vi "Get Position.vi"(8 "error in":errorcluster, 11 "Cell Context in":refnum<class "Cell Context.lvclass">) -> (0 "error out":errorcluster, 2 "Position":cluster{"Row":i32, "Column":i32}, 3 "Cell Context out":refnum<class "Cell Context.lvclass">)   [LabVIEW 2023, in "SourceGrid.lvlib" / "Cell Context.lvclass"]
uses:
  Cell Context.lvclass
  Cell Context.lvclass/Cell Context.ctl
  D:/git/Sourcegrid-LabVIEW/dll/SourceGrid.dll
  dll/SourceGrid.dll
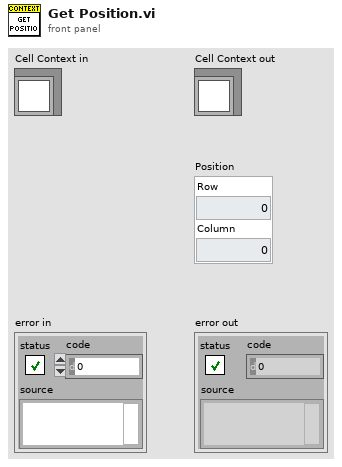
[diagram p1: front panel]
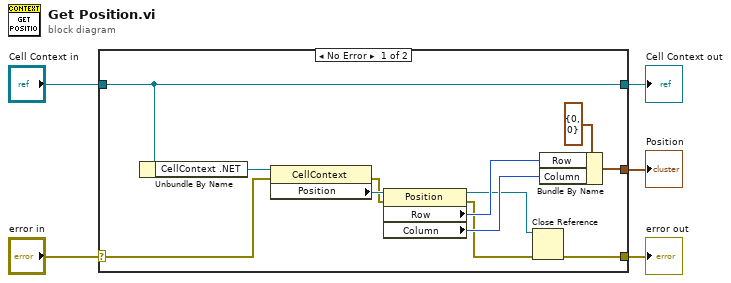
[diagram p0: block diagram]
diagram:
  n1 = case shown="No Error" "error in" {
    selector: "error in" -> [w16 w18]
    tunnel: [w7 w18] -> w4
    tunnel: [w17 w19] -> w2
    tunnel: "Cell Context in" -> [w17 w19]
    tunnel: [w13 _] -> w1
    frame No Error {
      n2 = Unbundle By Name(w17) -> ("CellContext .NET"=w8:refnum<k24>)
      n3 = property class="CellContext"(reference=w8, error in=w16) -> (error out=w9:errorcluster, "Position"=w15:refnum<k24>)  [unwired: 1 out]
      n4 = property class="Position"(reference=w15, error in=w9) -> (reference out=w6:refnum<k24>, error out=w10:errorcluster, "Row"=w12:i32, "Column"=w11:i32)
      n5 = Close Reference(reference=w6, error in (no error)=w10) -> (error out=w7:errorcluster)
      n6 = Bundle By Name(cluster=cluster{"Row":i32, "Column":i32} {"Row"=0, "Column"=0} ("Position 2"), "Row"=w12, "Column"=w11) -> (w13:cluster{"Row":i32, "Column":i32})
    }
    frame Error {
    }
  }
  "error out" <- w4
  "Cell Context out" <- w2
  "Position" <- w1
